vi "MTM2_getNextSample_powerStatus.vi"(8 "error in (no error)":errorcluster, 11 "powerStatus_Ctl":T1={"voltages[16]"=[0.0, 0.0, 0.0, 0.0, 0.0, 0.0, 0.0, 0.0, 0.0, 0.0, 0.0, 0.0, 0.0, 0.0, 0.0, 0.0], "currents[16]"=[0.0, 0.0, 0.0, 0.0, 0.0, 0.0, 0.0, 0.0, 0.0, 0.0, 0.0, 0.0, 0.0, 0.0, 0.0, 0.0], "onOff[16]"=[FALSE, FALSE, FALSE, FALSE, FALSE, FALSE, FALSE, FALSE, FALSE, FALSE, FALSE, FALSE, FALSE, FALSE, FALSE, FALSE], "states[16]"=[0, 0, 0, 0, 0, 0, 0, 0, 0, 0, 0, 0, 0, 0, 0, 0]}) -> (0 "error out":errorcluster, 2 "function return":i32, 3 "powerStatus_Ctl out":T1)   [LabVIEW 2018, in "SALLV_MTM2.lvlib"]
doc: "int MTM2_shm_getNextSample_powerStatusLV(MTM2_powerStatusLV *powerStatus_Ctl );"
uses:
  SALLV_MTM2.lvlib
  DataTypes/powerStatus.ctl
  SALLV_MTM2.so
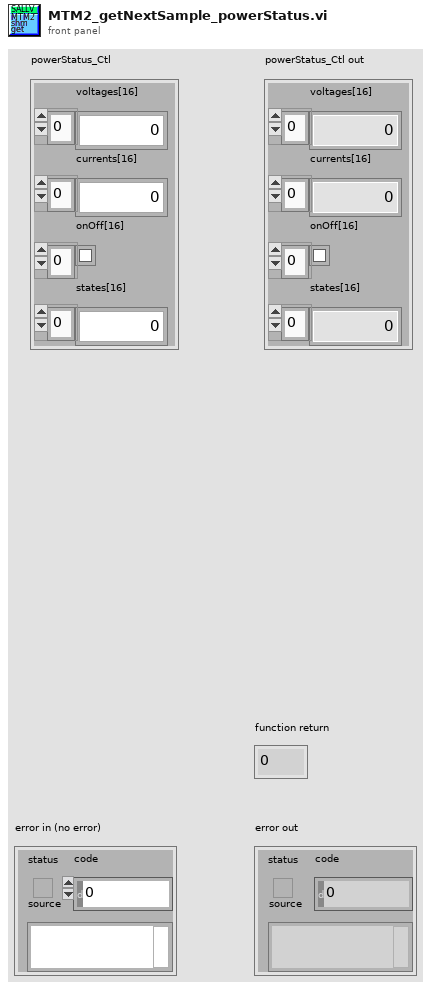
[diagram p1: front panel]
types:
  T1 = typedef "SALLV_MTM2.lvlib/powerStatus.ctl" = cluster{"voltages[16]":dbl[], "currents[16]":dbl[], "onOff[16]":bool[], "states[16]":u32[]}
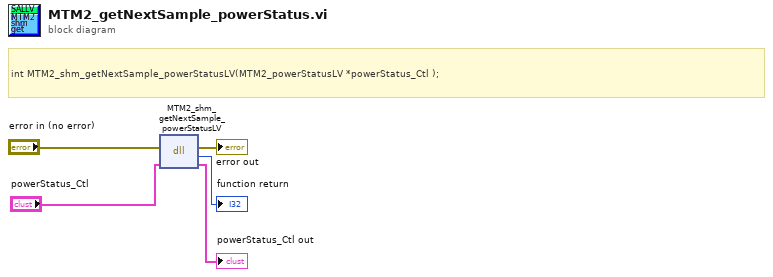
[diagram p0: block diagram]
diagram:
  # "int MTM2_shm_getNextSample_powerStatusLV(MTM2_powerStatusLV *powerStatus_Ctl );"
  n1 = dll-call lib="home/ttsai/Document/salApiMTM2/SALLV_MTM2/SALLV_MTM2.*" fn="MTM2_shm_getNextSample_powerStatusLV"(error in="error in (no error)", "powerStatus_Ctl"="powerStatus_Ctl") -> (error out=→"error out":errorcluster, →"function return":i32, "powerStatus_Ctl"=→"powerStatus_Ctl out":T1)  [unwired: 2 in, 1 out]
